vi "RichToFlatcif_template_GetResultRequest.vi"(5 "OutputClusterType":T1, 11 "InputCluster":T2) -> (3 "OutputCluster":T1)   [LabVIEW 2021, in "Template_server.lvlib"]
uses:
  Template_server.lvlib
  cif_template_GetResultRequest.ctl
  cif_template_GetResultRequest_Flat.ctl
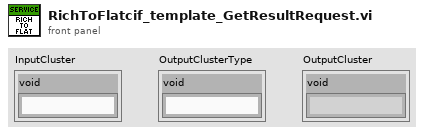
[diagram p1: front panel]
types:
  T1 = typedef "Template_server.lvlib/cif_template_GetResultRequest_Flat.ctl" = cluster{"void":string}
  T2 = typedef "Template_server.lvlib/cif_template_GetResultRequest.ctl" = cluster{"void":string}
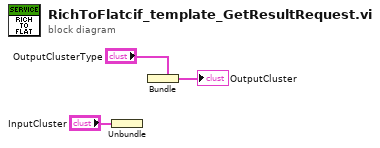
[diagram p0: block diagram]
diagram:
  n1 = Unbundle "Unbundle"("InputCluster") -> ()  [unwired: 1 out]
  n2 = Bundle "Bundle"(cluster="OutputClusterType") -> (→"OutputCluster":T1)  [unwired: 1 in]
